vi "Rysowanie prostej pod zadanym kątem.vi"(9 "Parametry prostej":T1={"Położenie końca"={"Pixel x"=0, "Pixel y"=0}, "Kolor"=0, "Długość [px]"=26, "Kąt/azymut"=2.0, "Interpretacją kąta ustawienia strzałki"=enum."Kąt trygonometryczny", "Grubość"=2}, 10 "Właściwości mapy":T2={"Przesunięcie mapy"={"X"=0, "Y"=0}, "Zoom"=1.0, "Długość piksela w metrach"=0.19634281539316645}, 11 "Mapa terenu":picture) -> (3 "Mapa z narysowaną prostą":picture)   [LabVIEW 2012, in "Biblioteka moduł map v3.lvlib" / "Obsługa grafiki mapy.lvlib"]
doc: "Zadaniem pliku jest dorysowanie do mapy terenu fragmentu prostej o zadanym położeniu końcowym i długości ustawionej pod wskazanym kątem. Kąt pod ktorym ustawiona jest prosta może oznaczać kąt trygonometryczny lub azymut."
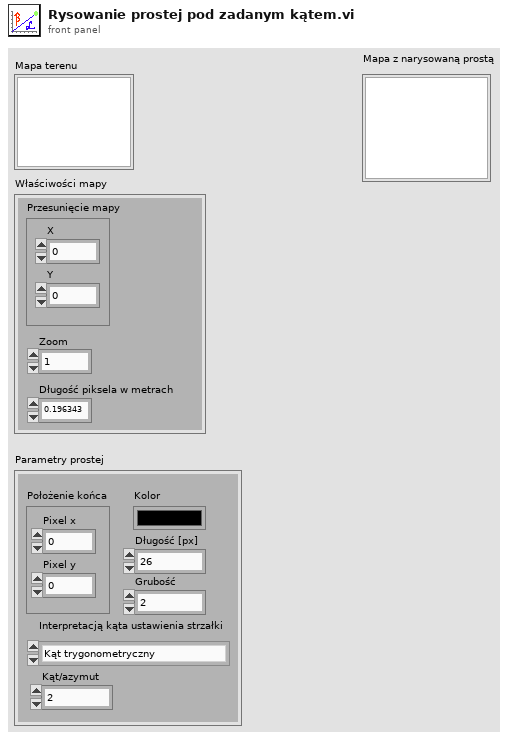
[diagram p1: front panel]
types:
  T1 = cluster{"Położenie końca":cluster{"Pixel x":i16, "Pixel y":i16}, "Kolor":u32, "Długość [px]":u32, "Kąt/azymut":dbl, "Interpretacją kąta ustawienia strzałki":enum16{"Kąt trygonometryczny", "Azymut"}, "Grubość":u32}
  T2 = cluster{"Przesunięcie mapy":cluster{"X":i16, "Y":i16}, "Zoom":dbl, "Długość piksela w metrach":dbl}
  T3 = cluster{"Położenie":cluster{"Pixel x":i16, "Pixel y":i16}, "Kolor punktu":u32, "Rozmiar punktu":u32, "Nazwa punktu":string}
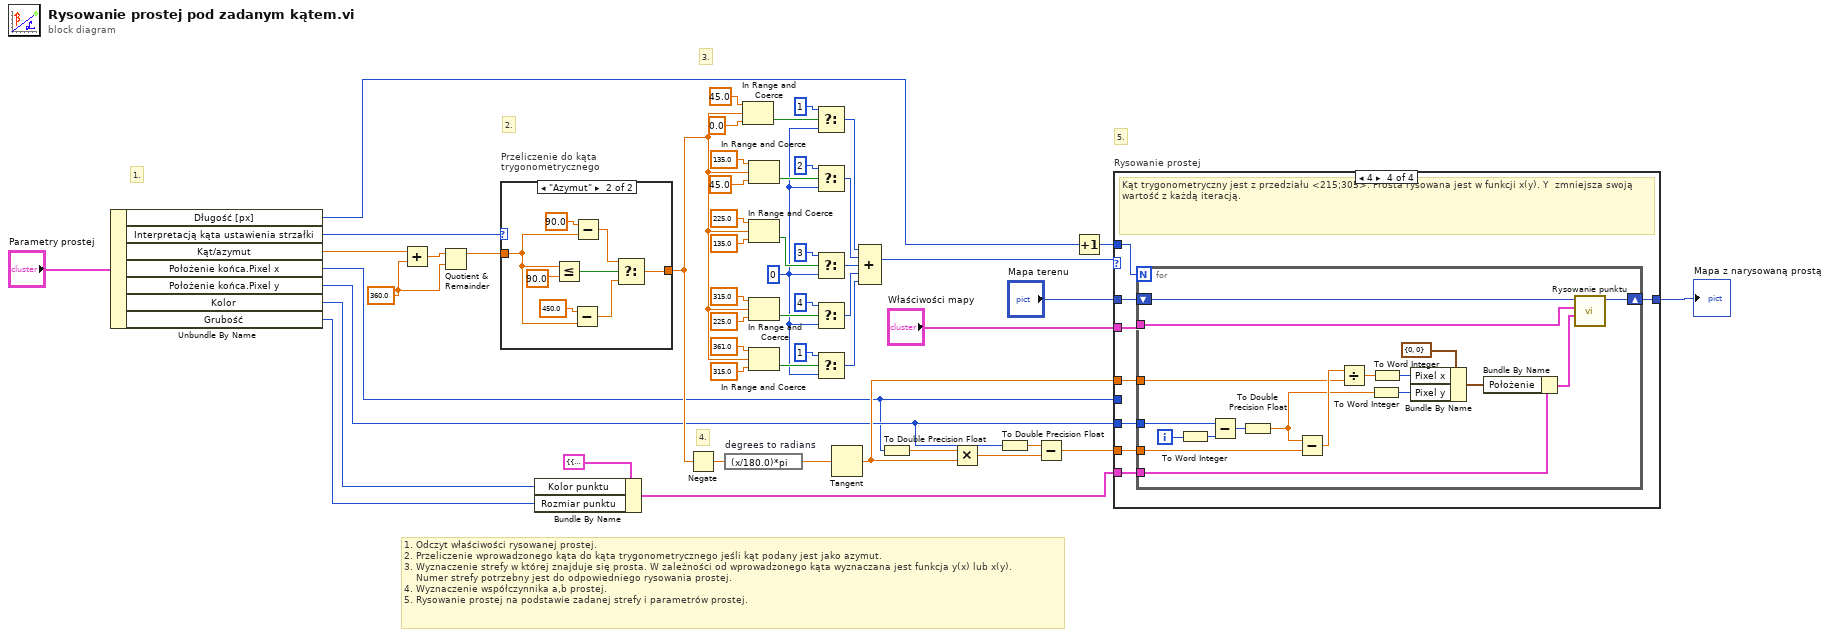
[diagram p0: block diagram]
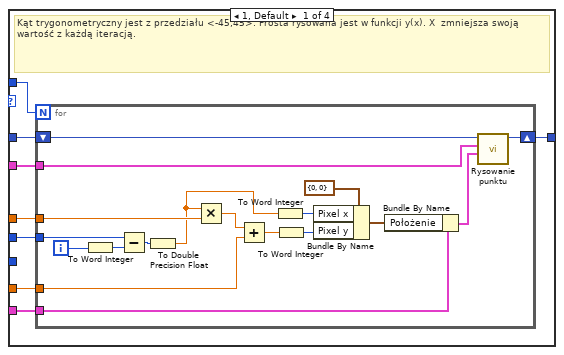
[diagram p2: hidden frame]
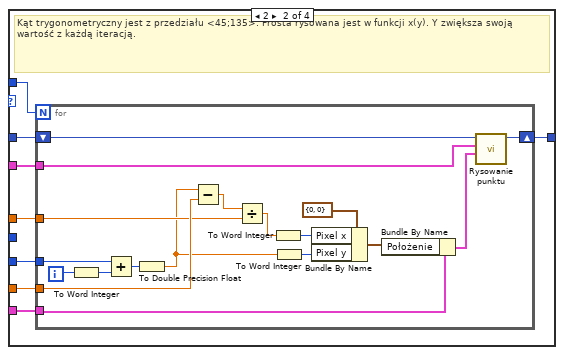
[diagram p3: hidden frame]
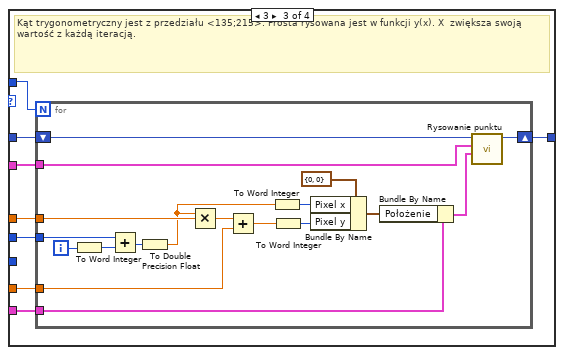
[diagram p4: hidden frame]
diagram:
  w2 = 360.0 ("y")
  w24 = i8 0 ("f")
  # "1. Odczyt właściwości rysowanej prostej.\n2. Przeliczenie wprowadzonego kąta do kąta trygonometrycznego jeśli kąt podany jest jako azymut.\n3. Wyznaczenie strefy w której znajduje się prosta. W zależności od wprowadzonego kąta wyznaczana jest funkcja y(x) lub x(y).\n    Numer strefy potrzebny jest do odpowiedniego rysowania prostej.\n4. Wyznaczenie współczynnika a,b prostej.\n5. Rysowanie prostej na podstawie zadanej strefy i parametrów prostej."
  # "5."
  # "4."
  # "3."
  # "2."
  # "1."
  n1 = Unbundle By Name("Parametry prostej") -> ("Długość [px]"=w10:u32, "Interpretacją kąta ustawienia strzałki"=w9:enum16{"Kąt trygonometryczny", "Azymut"}, "Kąt/azymut"=w4:dbl, "Położenie końca.Pixel x"=w7:i16, "Położenie końca.Pixel y"=w8:i16, "Kolor"=w6:u32, "Grubość"=w5:u32)
  n2 = Add(x=w4, y=w2) -> (x+y=w3:dbl)
  n3 = Quotient & Remainder(x=w3, y=w2) -> (x-y*floor(x/y)=w1:dbl)  [unwired: 1 out]
  n4 = case "Przeliczenie do kąta trygonometrycznego" shown="\"Azymut\"" w9 {
    tunnel: [w53 w55] -> w14
    tunnel: w1 -> [w53 w54]
    frame "Kąt trygonometryczny", Default {
    }
    frame "Azymut" {
      n5 = Less Or Equal?(x=w54, y=90.0) -> (x <= y?=w59:bool)
      n6 = Subtract(x=450.0, y=w54) -> (x-y=w58:dbl)
      n7 = Subtract(x=90.0, y=w54) -> (x-y=w56:dbl)
      n8 = Select(t=w56, s=w59, f=w58) -> (s? t:f=w55:dbl)
    }
  }
  n9 = Bundle By Name(cluster=T3 {"Położenie"={"Pixel x"=0, "Pixel y"=0}, "Kolor punktu"=0, "Rozmiar punktu"=2, "Nazwa punktu"=""} ("Punkt na mapie"), "Kolor punktu"=w6, "Rozmiar punktu"=w5) -> (w11:T3)
  n10 = Negate(x=w14) -> (-x=w48:dbl)
  n11 = expression code="(x/180.0)*pi" "degrees to radians"(w48) -> (w50:dbl)
  n12 = In Range and Coerce(upper limit=45.0, x=w14, lower limit=0.0) -> (In Range?=w30:bool)  [unwired: 1 out]
  n13 = In Range and Coerce(upper limit=135.0, x=w14, lower limit=45.0) -> (In Range?=w26:bool)  [unwired: 1 out]
  n14 = In Range and Coerce(upper limit=225.0, x=w14, lower limit=135.0) -> (In Range?=w27:bool)  [unwired: 1 out]
  n15 = In Range and Coerce(upper limit=315.0, x=w14, lower limit=225.0) -> (In Range?=w28:bool)  [unwired: 1 out]
  n16 = In Range and Coerce(upper limit=361.0, x=w14, lower limit=315.0) -> (In Range?=w29:bool)  [unwired: 1 out]
  n17 = Select(t=i8 1, s=w30, f=w24) -> (s? t:f=w19:i8)
  n18 = Select(t=i8 2, s=w26, f=w24) -> (s? t:f=w18:i8)
  n19 = Select(t=i8 3, s=w27, f=w24) -> (s? t:f=w17:i8)
  n20 = Select(t=i8 4, s=w28, f=w24) -> (s? t:f=w16:i8)
  n21 = Select(t=i8 1, s=w29, f=w24) -> (s? t:f=w15:i8)
  n22 = Tangent(1:w50) -> (0:w45:dbl)
  n23 = Compound Arithmetic op=ADD(w19, w18, w17, w16, w15) -> (w13:i8)
  n24 = To Double Precision Float(number=w7) -> (double precision float=w46:dbl)
  n25 = Multiply(x=w46, y=w45) -> (x*y=w52:dbl)
  n26 = To Double Precision Float(number=w8) -> (double precision float=w47:dbl)
  n27 = Subtract(x=w47, y=w52) -> (x-y=w51:dbl)
  n28 = Increment(x=w10) -> (x+1=w49:u32)
  n29 = case "Rysowanie prostej" shown="4" w13 {
    tunnel: "Mapa terenu" -> [w69 w94 w118 w141]
    tunnel: w45 -> [w68 w93 w119 w144]
    tunnel: w51 -> [w67 w92 w120 w145]
    tunnel: [w66 w91 w117 w147] -> w44
    tunnel: w49 -> [w65 w95 w121 w146]
    tunnel: "Właściwości mapy" -> [w64 w90 w116 w143]
    tunnel: w7 -> [w63 _ w115 _]
    tunnel: w8 -> [_ w89 _ w142]
    tunnel: w11 -> [w62 w88 w114 w140]
    frame 1, Default {
      # "Kąt trygonometryczny jest z przedziału <-45;45>. Prosta rysowana jest w funkcji y(x). X  zmniejsza swoją wartość z każdą iteracją."
      n30 = for {
        N: w65 -> [_]
        shift-right: [w82] -> w66
        shift-left: w69 -> [w83]
        tunnel: w68 -> [w87]
        tunnel: w67 -> [w85]
        tunnel: w64 -> [w81]
        tunnel: w63 -> [w80]
        tunnel: w62 -> [w78]
        i -> [w70]
        n31 = To Word Integer(number=w70) -> (16bit integer=w71:i16)
        n32 = Subtract(x=w80, y=w71) -> (x-y=w84:i16)
        n33 = To Double Precision Float(number=w84) -> (double precision float=w73:dbl)
        n34 = Multiply(x=w73, y=w87) -> (x*y=w86:dbl)
        n35 = Add(x=w86, y=w85) -> (x+y=w72:dbl)
        n36 = To Word Integer(number=w73) -> (16bit integer=w76:i16)
        n37 = To Word Integer(number=w72) -> (16bit integer=w75:i16)
        n38 = Bundle By Name(cluster=cluster{"Pixel x":i16, "Pixel y":i16} {"Pixel x"=0, "Pixel y"=0} ("Położenie"), "Pixel x"=w76, "Pixel y"=w75) -> (w74:cluster{"Pixel x":i16, "Pixel y":i16})
        n39 = Bundle By Name(cluster=w78, "Położenie"=w74) -> (w79:T3)
        n40 = call "Rysowanie punktu.vi"("Punkt na mapie"=w79, "Właściwości mapy"=w81, "Mapa terenu"=w83) -> ("Mapa z wprowadzonym punktem"=w82:picture)  [unwired: 8 in]
      }
    }
    frame 2 {
      # "Kąt trygonometryczny jest z przedziału <45;135>. Prosta rysowana jest w funkcji x(y). Y zwiększa swoją wartość z każdą iteracją."
      n41 = for {
        N: w95 -> [_]
        shift-right: [w109] -> w91
        shift-left: w94 -> [w108]
        tunnel: w93 -> [w111]
        tunnel: w92 -> [w112]
        tunnel: w90 -> [w107]
        tunnel: w89 -> [w106]
        tunnel: w88 -> [w104]
        i -> [w96]
        n42 = To Word Integer(number=w96) -> (16bit integer=w97:i16)
        n43 = Add(x=w106, y=w97) -> (x+y=w110:i16)
        n44 = To Double Precision Float(number=w110) -> (double precision float=w99:dbl)
        n45 = Subtract(x=w99, y=w112) -> (x-y=w113:dbl)
        n46 = Divide(x=w113, y=w111) -> (x/y=w98:dbl)
        n47 = To Word Integer(number=w98) -> (16bit integer=w102:i16)
        n48 = To Word Integer(number=w99) -> (16bit integer=w101:i16)
        n49 = Bundle By Name(cluster=cluster{"Pixel x":i16, "Pixel y":i16} {"Pixel x"=0, "Pixel y"=0} ("Położenie"), "Pixel x"=w102, "Pixel y"=w101) -> (w100:cluster{"Pixel x":i16, "Pixel y":i16})
        n50 = Bundle By Name(cluster=w104, "Położenie"=w100) -> (w105:T3)
        n51 = call "Rysowanie punktu.vi"("Punkt na mapie"=w105, "Właściwości mapy"=w107, "Mapa terenu"=w108) -> ("Mapa z wprowadzonym punktem"=w109:picture)  [unwired: 8 in]
      }
    }
    frame 3 {
      # "Kąt trygonometryczny jest z przedziału <135;215>. Prosta rysowana jest w funkcji y(x). X  zwiększa swoją wartość z każdą iteracją."
      n52 = for {
        N: w121 -> [_]
        shift-right: [w134] -> w117
        shift-left: w118 -> [w135]
        tunnel: w119 -> [w139]
        tunnel: w120 -> [w137]
        tunnel: w116 -> [w133]
        tunnel: w115 -> [w132]
        tunnel: w114 -> [w131]
        i -> [w122]
        n53 = To Word Integer(number=w122) -> (16bit integer=w123:i16)
        n54 = Add(x=w132, y=w123) -> (x+y=w136:i16)
        n55 = To Double Precision Float(number=w136) -> (double precision float=w126:dbl)
        n56 = Multiply(x=w126, y=w139) -> (x*y=w138:dbl)
        n57 = Add(x=w138, y=w137) -> (x+y=w125:dbl)
        n58 = To Word Integer(number=w126) -> (16bit integer=w128:i16)
        n59 = To Word Integer(number=w125) -> (16bit integer=w127:i16)
        n60 = Bundle By Name(cluster=cluster{"Pixel x":i16, "Pixel y":i16} {"Pixel x"=0, "Pixel y"=0} ("Położenie"), "Pixel x"=w128, "Pixel y"=w127) -> (w124:cluster{"Pixel x":i16, "Pixel y":i16})
        n61 = Bundle By Name(cluster=w131, "Położenie"=w124) -> (w130:T3)
        n62 = call "Rysowanie punktu.vi"("Punkt na mapie"=w130, "Właściwości mapy"=w133, "Mapa terenu"=w135) -> ("Mapa z wprowadzonym punktem"=w134:picture)  [unwired: 8 in]
      }
    }
    frame 4 {
      # "Kąt trygonometryczny jest z przedziału <215;305>. Prosta rysowana jest w funkcji x(y). Y  zmniejsza swoją wartość z każdą iteracją."
      n63 = for {
        N: w146 -> [_]
        shift-right: [w160] -> w147
        shift-left: w141 -> [w159]
        tunnel: w144 -> [w162]
        tunnel: w145 -> [w163]
        tunnel: w143 -> [w158]
        tunnel: w142 -> [w157]
        tunnel: w140 -> [w156]
        i -> [w149]
        n64 = To Word Integer(number=w149) -> (16bit integer=w148:i16)
        n65 = Subtract(x=w157, y=w148) -> (x-y=w161:i16)
        n66 = To Double Precision Float(number=w161) -> (double precision float=w150:dbl)
        n67 = Subtract(x=w150, y=w163) -> (x-y=w164:dbl)
        n68 = Divide(x=w164, y=w162) -> (x/y=w153:dbl)
        n69 = To Word Integer(number=w150) -> (16bit integer=w151:i16)
        n70 = To Word Integer(number=w153) -> (16bit integer=w152:i16)
        n71 = Bundle By Name(cluster=cluster{"Pixel x":i16, "Pixel y":i16} {"Pixel x"=0, "Pixel y"=0} ("Położenie"), "Pixel x"=w152, "Pixel y"=w151) -> (w155:cluster{"Pixel x":i16, "Pixel y":i16})
        n72 = Bundle By Name(cluster=w156, "Położenie"=w155) -> (w154:T3)
        n73 = call "Rysowanie punktu.vi"("Punkt na mapie"=w154, "Właściwości mapy"=w158, "Mapa terenu"=w159) -> ("Mapa z wprowadzonym punktem"=w160:picture)  [unwired: 8 in]
      }
    }
  }
  "Mapa z narysowaną prostą" <- w44
